vi "SFID.vi"() -> (0 "error out":errorcluster)   [LabVIEW 2022 SP3]
uses:
  Sub_vis/Upload Data.ctl
  Globals/Meas_global.vi
panel:
  out "No Of samples":dbl
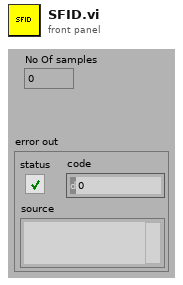
[diagram p1: front panel]
types:
  T1 = typedef "Setup.ctl" = enum16{"Run Program", "Show Setup", "Save Current Setup", "Setup Front Panel"}
  T2 = typedef "Upload Data.ctl" = enum16{"Voltage Array", "Time Trace Cluster"}
  T3 = typedef "Analysis_info_cluster.ctl" = cluster{"Colour":u32, "Inst type":T4, "Inst name":string, "Symbol":string, "Code name":string, "Extra Info":string, "Inst Array":T5, "Extra Titles":string[], "Extra Values":string[], "U":dbl, "u^2":dbl, "u^3":dbl, "u^4":dbl, "Skew_u":dbl, "Kurt_u":dbl, "Sd Error in Mean":dbl, "% u'/U":dbl, "X":dbl, "Y":dbl, "Z":dbl, "Timescale integral Estimate":dbl, "Sd Error in Variance":dbl, "Calib File":path, "Calib Constants":dbl[], "Output Position":bool, "Stats":enum16{"None", "Basic", "Full"}, "Av Sampling Rate":dbl, "Av No of Samples":dbl, "Total Meas Time (s)":dbl, "ADAM Ch Name":string, "Max value":dbl, "Min value":dbl, "Req Sample Rate Hz":dbl, "Sync Delay Time (s)":dbl, "Ch No":i16, "Device":string, "Use Latest Calib":bool, "Port":string, "Metadata Ch Names":string[], "Metadata Ch Values":string[], "Label":string}
  T4 = typedef "Inst_type.ctl" = enum16{"Raw voltage", "Raw with zero offsetting", "Propeller anemometer", "Pressure Transducer", "Pitot-static tube", "Hot wire", "Cross wire 1", "Cross wire 2", "Generic Linear", "Generic Polynomial", "Generic BackPoly", "Fast FID", "Thermocouple", "Cold wire", "Pulsed Wire", "LDA Vel", "LDA Tran time", "LDA Arr time", "Microphone"}
  T5 = typedef "Instrument_Array.ctl" = enum16{"PWA", "LDA", "Analogue"}
  T6 = typedef "Rendezvous RefNum" = refnum<k1>
  T7 = typedef "Device ID port info.ctl" = cluster{"Ch No":i16[], "Req Sampling Rate":dbl[], "Port":string, "Index":i32[]}
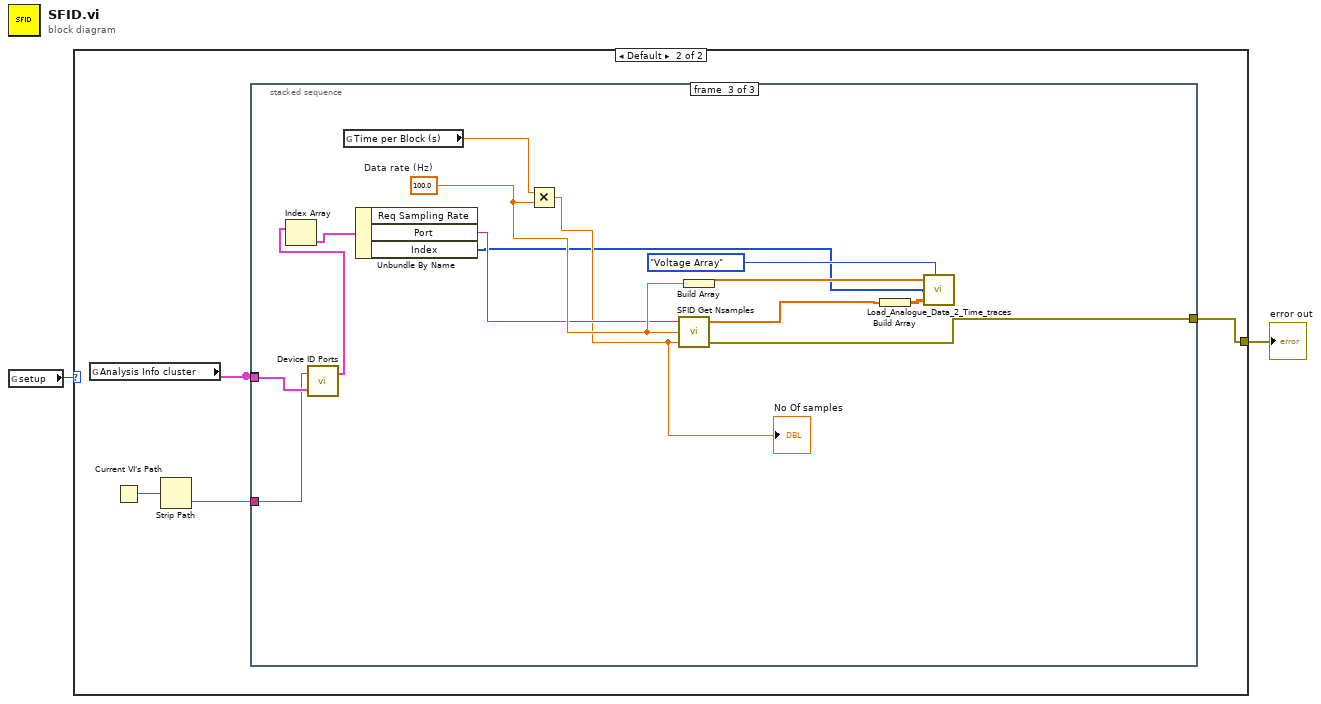
[diagram p0: block diagram]
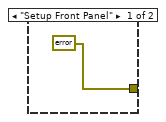
[diagram p2: hidden frame]
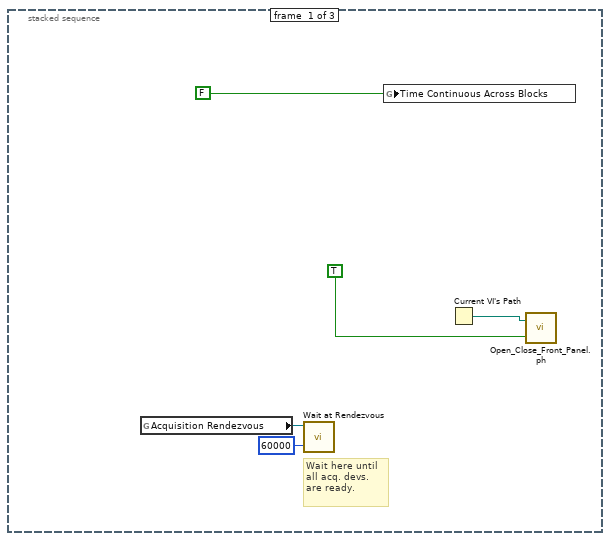
[diagram p3: hidden frame]
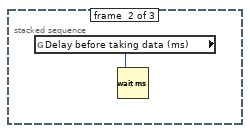
[diagram p4: hidden frame]
diagram:
  n1 = global read "Meas_global.vi" "setup"() -> (w2:T1)
  n2 = case shown="Default" w2 {
    tunnel: [errorcluster {"status"=FALSE, "code"=0, "source"=""} ("error out") w7] -> w1
    frame "Setup Front Panel" {
    }
    frame Default {
      n3 = global read "Meas_global.vi" "Analysis Info cluster"() -> (w5:T3[])
      n4 = Current VI's Path() -> (path=w6:path)
      n5 = Strip Path(path=w6) -> (name=w4:string)  [unwired: 1 out]
      n6 = stacked-sequence {
        tunnel: w5 -> [_ _ _]
        tunnel: [_ _ w22] -> w7
        tunnel: w5 -> [_ _ w18]
        tunnel: w4 -> [_ _ w17]
        frame #0 {
          # "Wait here until all acq. devs. are ready."
          n7 = global read "Meas_global.vi" "Acquisition Rendezvous"() -> (w9:T6)
          n8 = call <vilib>:"Wait at Rendezvous.vi"("ms timeout (-1)"=60000, "rendezvous"=w9) -> ()  [unwired: 3 in, 3 out]
          n9 = global write "Meas_global.vi" "Time Continuous Across Blocks"(FALSE ("Time Continuous across Blocks")) -> ()
          n10 = Current VI's Path() -> (path=w12:path)
          n11 = call "Open_Close_Front_Panel.ph.vi"("openWindow (T)"=TRUE ("Front Panel Window:Open"), "VI path"=w12) -> ()  [unwired: 1 in, 1 out]
        }
        frame #1 {
          n12 = global read "Meas_global.vi" "Delay before taking data (ms)"() -> (w13:u32)
          n13 = Wait (ms)(milliseconds to wait=w13) -> ()  [unwired: 1 out]
        }
        frame #2 {
          w21 = 100.0  # Data rate (Hz)
          n14 = call "Device ID Ports.vi"("Analysis Info cluster"=w18, "Device ID"=w17) -> ("Device port info"=w16:T7[])  [unwired: 1 out]
          n15 = Index Array(array=w16) -> (element=w26:T7)  [unwired: 1 in]
          n16 = global read "Meas_global.vi" "Time per Block (s)"() -> (w27:dbl)
          n17 = Unbundle By Name(w26) -> ("Port"=w20:string, "Index"=w15:i32[])  [unwired: 1 out]
          n18 = Multiply(x=w27, y=w21) -> (x*y=w19:dbl)
          "No Of samples" <- w19
          n19 = call "SFID Get Nsamples.vi"("N samples"=w19, "Data rate (Hz) In"=w21, "COM port"=w20) -> ("Error out"=w22:errorcluster, "Voltage array out"=w14:sgl[])  [unwired: 1 out]
          n20 = Build Array(w21) -> (w25:dbl[])
          n21 = Build Array(w14) -> (w24:sgl[][])
          n22 = call "Load_Analogue_Data_2_Time_traces.vi"("Sampling Rate (Hz)"=w25, "Mode"=Upload_Data."Voltage Array", "Index"=w15, "Voltage Array"=w24) -> ()  [unwired: 3 in]
        }
      }
    }
  }
  "error out" <- w1
